vi "config UI.vi"() -> ()   [LabVIEW 2017, in "ScaleAndLimitModule editor node.lvclass"]
doc: "All child modules share this same UI. The UI allows for the configuration of Channels, Parameters, and Error Handling."
uses:
  ScaleAndLimitModule editor node.lvclass
  <vilib>/NI/Configuration Framework/Node/NodeRef.ctl
  <vilib>/NI/Configuration Framework/Node/NISE_CEF_Node.lvclass
  <vilib>/NI/AMC/Message Queue.ctl
  <vilib>/NI/AMC/Message.ctl
  <vilib>/NI/Tools/Keyed Array/KeyedArray.ctl
  <vilib>/NI/Configuration Framework/Node/UserEventRef.ctl
  <vilib>/NI/Configuration Framework/Controls/EventCluster.ctl
  <vilib>/NI/DCAF/Tag Editor Core/control module/configuration/error classification setting.ctl
  <vilib>/NI/Tag Bus Module Framework/runtime/error classification.ctl
  <vilib>/NI/Configuration Framework/Node/RefreshUIEvent.ctl
  <vilib>/NI/Configuration Framework/Node/CacheState.ctl
  <vilib>/NI/Configuration Framework/Node/StopEvent.ctl
  <vilib>/NI/Configuration Framework/Node/NodeChangeEvent.ctl
  <vilib>/NI/DCAF/Tag Editor Core/Table API/Available Tag Menu/channel action event.ctl
  <vilib>/NI/DCAF/Tag Editor Core/Table API/Available Tag Menu/dialog output action.ctl
  <vilib>/NI/Tag Bus Module Framework/channel/TBM channel.lvclass
  <vilib>/NI/Tag Bus/tag/tag descriptor.lvclass
  <vilib>/NI/DCAF/Tag Editor Core/Table API/Table Manager/Call Back Ref Type Def.ctl
  <vilib>/NI/DCAF/Tag Editor Core/Configuration Editor/Classes/Engine Parent/Engine Parent Editor Node.lvclass
  <vilib>/NI/DCAF/Tag Editor Core/Configuration Editor/Classes/Module editor node/module editor node.lvclass
  C:/Program Files (x86)/National Instruments/LabVIEW 2017/vi.lib/NI/Configuration Framework/serializable node/NISE_CEF_serializable node.lvclass
  <vilib>/NI/DCAF/Tag Editor Core/Table API/Table Manager/references.ctl
  <vilib>/NI/DCAF/Tag Editor Core/Table API/Table Manager/Menu Definition.ctl
  <vilib>/NI/DCAF/Tag Editor Core/Table API/Table Manager/Menu Options.ctl
  <vilib>/NI/DCAF/Tag Editor Core/control module/configuration/control module configuration.lvclass
  C:/Program Files (x86)/National Instruments/LabVIEW 2017/vi.lib/NI/Configuration Framework/serializable configuration/NISE_CEF_serializable configuration.lvclass
  <vilib>/NI/DCAF/Tag Editor Core/control module/editor node/control module editor.lvclass
  module/configuration/ScaleAndLimitModule configuration.lvclass
  C:/Program Files (x86)/National Instruments/LabVIEW 2017/vi.lib/NI/DCAF/Tag Editor Core/control module/configuration/control module configuration.lvclass
  C:/Program Files (x86)/National Instruments/LabVIEW 2017/vi.lib/NI/Tag Bus Module Framework/module configuration/TBM module configuration.lvclass
  module/configuration/ScaleAndLimitModule configuration.lvclass/ScaleAndLimitModule configuration.ctl
  <vilib>/NI/DCAF/Tag Editor Core/control module/configuration/control module configuration.lvclass/control module configuration.ctl
  <vilib>/NI/Configuration Framework/serializable configuration/NISE_CEF_serializable configuration.lvclass/NISE_CEF_serializable configuration.ctl
  <vilib>/NI/Tag Bus Module Framework/channel/channel classification.ctl
  module/configuration/Read ScaleAndLimitConfig.vi
  module/configuration/Write ScaleAndLimitConfig.vi
  <vilib>/NI/DCAF/Tag Editor Core/control module/configuration/Write error classifications.vi
  <vilib>/NI/Tag Bus Module Framework/module configuration/TBM module configuration.lvclass
  <vilib>/NI/DCAF/Tag Editor Core/Configuration Editor/Classes/Module editor node/Read Module Configuration.vi
  <vilib>/NI/DCAF/Tag Editor Core/control module/editor node/read fixed channel configuration.vi
  <vilib>/Utility/LVClass/Get LV Class Name.vi
  <vilib>/NI/Configuration Framework/error generator/NISE_error generator.vi
  <vilib>/NI/DCAF/Tag Editor Core/Configuration Editor/Classes/Module editor node/Write Module Configuration.vi
  <vilib>/NI/Configuration Framework/serializable configuration/NISE_CEF_serializable configuration.lvclass
  <vilib>/NI/DCAF/Tag Editor Core/Table API/Listbox/Multi Column Listbox.lvclass
  <vilib>/NI/Configuration Framework/NISE_CEF_TreeControl.lvlib
  <vilib>/NI/DCAF/Tag Editor Core/Table API/Table Manager.lvlib
  <vilib>/NI/DCAF UI Toolkit/Controls/DCAF UI Elements.lvlib
  <vilib>/NI/Tools/Keyed Array/Tools_KeyedArray.lvlib
  <vilib>/NI/AMC/AMC.lvlib
  <vilib>/NI/DCAF/Tag Editor Core/Table API/Table Manager/Table Manager.lvclass
  <vilib>/NI/Tag Bus Module Framework/runtime/TBM module execution interface.lvclass
panel:
  in  "Enum":i32
  in  "user event out":refnum<user-event>
  in  "Top Level Tab Control":T1(tab)
  in  "Values":T2(array[cluster])
  in  "Channels Listbox":i32(listbox)
  in  "mapall":bool
  in  "mapwriters":bool
  in  "Parameters Listbox":i32(listbox)
  in  "error classifications":T3[](array[typedef])
  in  "node change":T5
  in  "stop event":T6
  in  "cache state":T7
  in  "refresh UI":T8
  in  "user event":T9
  in  "main queue":T10
  in  "node ref":T11
  # "Name                                       M                                 B                      High Limit                 Low Limit            Limits Enable"
  # "Y=M*(X-B)"
  # "0"
  # "5"
  # "10"
  # "15"
  # "(Single-Click to Edit)"
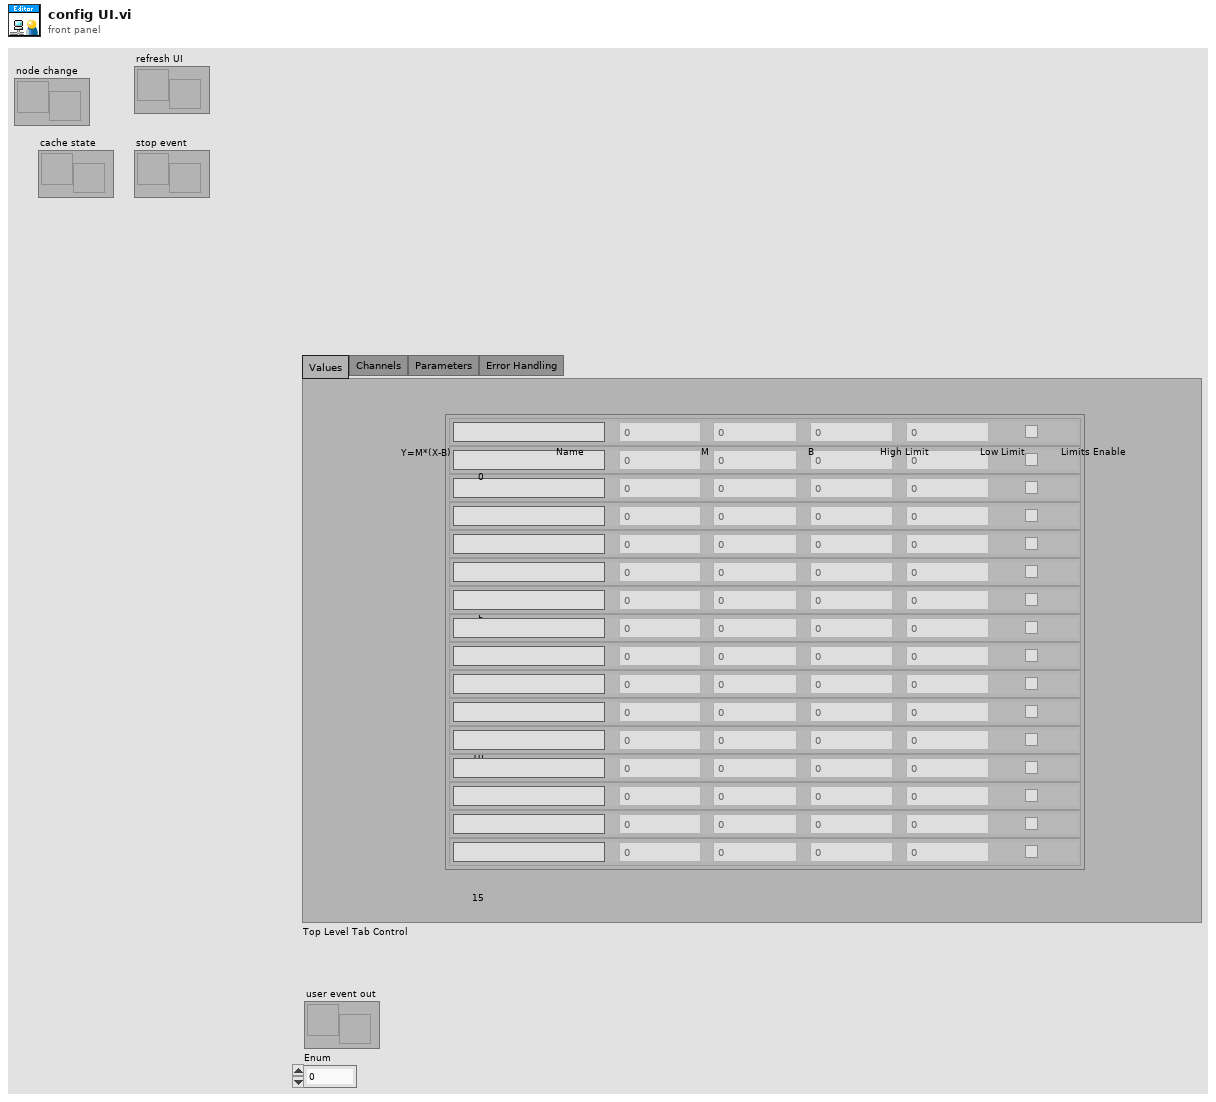
[diagram p1: front panel]
types:
  T1 = enum32{"Values", "Channels", "Parameters", "Error Handling"}
  T2 = cluster{"Name":string, "M":sgl, "B":i16, "HighLimit":sgl, "LowLimit":sgl, "LimitsEnabled":bool}[]
  T3 = typedef "control module configuration.lvclass/error classification setting.ctl" = cluster{"code":i32, "error classification":T4}
  T4 = typedef "TBM module execution interface.lvclass/error classification.ctl" = enum16{"unknown", "none", "trivial", "recoverable", "critical"}
  T5 = typedef "NISE_CEF_Node.lvclass/NodeChangeEvent.ctl" = refnum<user-event>
  T6 = typedef "NISE_CEF_Node.lvclass/StopEvent.ctl" = refnum<user-event>
  T7 = typedef "NISE_CEF_Node.lvclass/CacheState.ctl" = refnum<user-event>
  T8 = typedef "NISE_CEF_Node.lvclass/RefreshUIEvent.ctl" = refnum<user-event>
  T9 = typedef "NISE_CEF_Node.lvclass/UserEventRef.ctl" = refnum<user-event>
  T10 = typedef "AMC.lvlib/Message Queue.ctl" = refnum<queue>
  T11 = typedef "NISE_CEF_Node.lvclass/NodeRef.ctl" = refnum<data-value>
  T12 = typedef "Table Manager.lvlib/Table Manager.lvclass/Menu Definition.ctl" = cluster{"Menu Name":string, "Menu Options":T13}
  T13 = typedef "Table Manager.lvlib/Table Manager.lvclass/Menu Options.ctl" = enum16{"Always Show", "Show When Used", "Show When Empty"}
  T14 = typedef "Table Manager.lvlib/Table Manager.lvclass/references.ctl" = cluster{"stop event":T6, "refresh UI":T8, "cache state":T7, "node change":T5, "user event out":refnum<user-event>, "main queue":T10, "user event":T9}
  T15 = typedef "Table Manager.lvlib/Column.lvclass/Column Descriptor.ctl" = cluster{"name":string, "caption":string, "Column Type":T16, "Params":string, "AutoSizeMode":i32, "FillWeight":sgl, "MinWidth":u32, "tooltip":string, "Enum Reference":refnum<vi>, "Channel suffix":string, "Read Only":bool, "Call Back VI":T17, "DT Dependency":i32, "name dependency":i32, "data type":T18, "Custom Column":refnum<class "Column.lvclass">}
  T16 = typedef "Table Manager.lvlib/Column.lvclass/Column Type.ctl" = enum16{"String", "Mapping", "Enum", "Custom"}
  T17 = typedef "Table Manager.lvlib/Table Manager.lvclass/Call Back Ref Type Def.ctl" = refnum<vi>
  T18 = typedef "tag bus.lvlib/tag descriptor.lvclass/Data Type.ctl" = enum16{"Double", "Single", "I64", "I32", "I16", "I8", "U64", "U32", "U16", "U8", "Boolean", "String", "Array of Double", "Array of Single", "Array of I64", "Array of I32", "Array of I16", "Array of I8", "Array of U64", "Array of U32", "Array of U16", "Array of U8", "Array of Boolean", "Array of String"}
  T19 = typedef "Table Manager.lvlib/Table Manager.lvclass/object ref.ctl" = cluster{"engine":refnum<data-value>, "Node Ref":refnum<data-value>}
  T20 = typedef "Table Manager.lvlib/Table Manager.lvclass/Table Events.ctl" = cluster{"Menu Selection":refnum<user-event>}
  T21 = typedef "NISE_CEF_TreeControl.lvlib/EventCluster.ctl" = cluster{"command":string, "data":string}
  T22 = typedef "ScaleAndLimitInterface.lvlib/Configuration.ctl" = cluster{"Name":string, "M":dbl, "B":i16, "HighLimit":dbl, "LowLimit":dbl, "LimitsEnabled":bool}
  T23 = typedef "TBM channel.lvclass/channel classification.ctl" = enum16{"input data", "output data", "processing parameter", "processing result"}
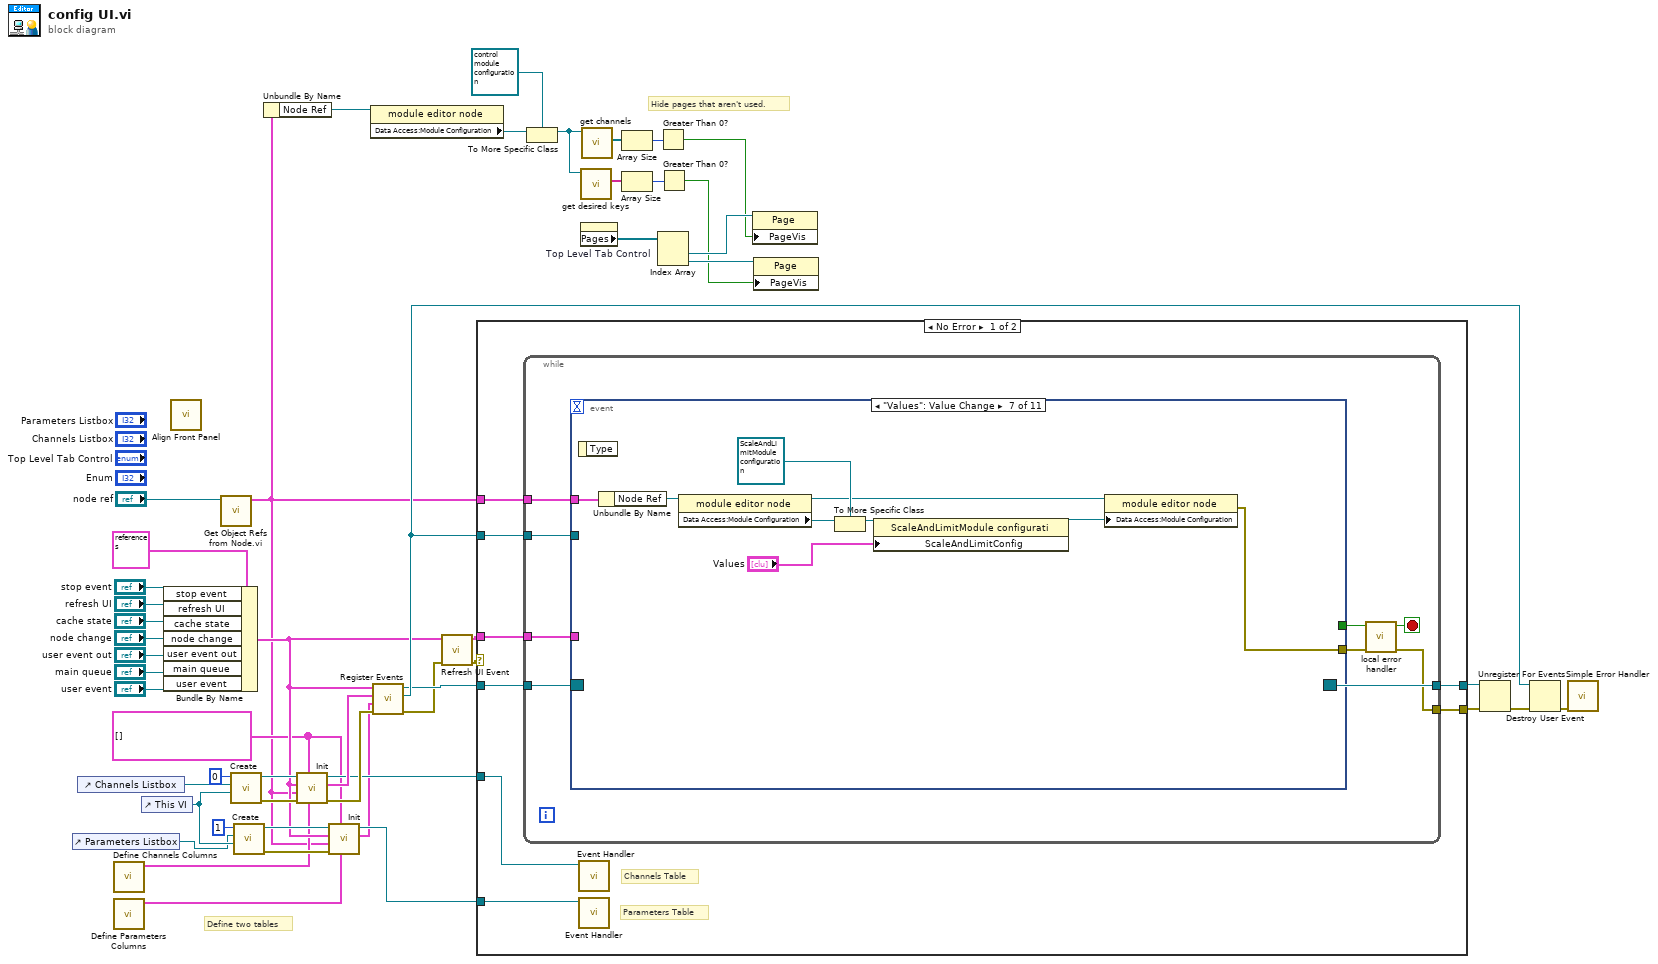
[diagram p0: block diagram]
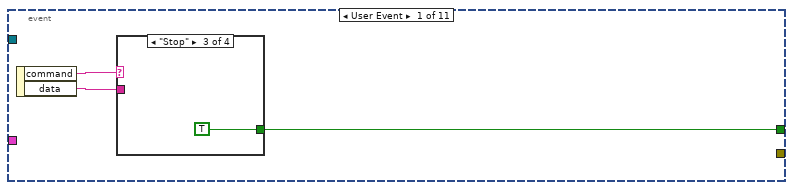
[diagram p2: hidden frame]
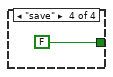
[diagram p5: hidden frame]
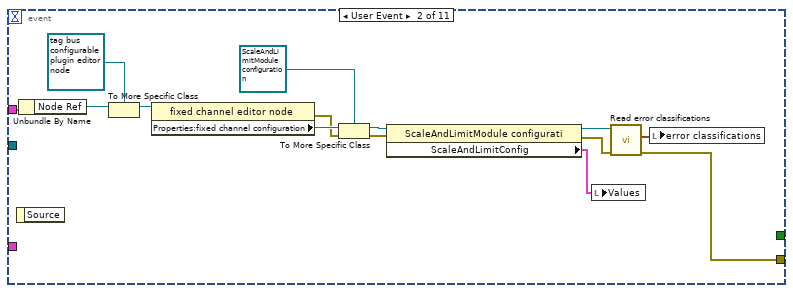
[diagram p6: hidden frame]
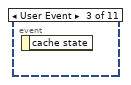
[diagram p7: hidden frame]
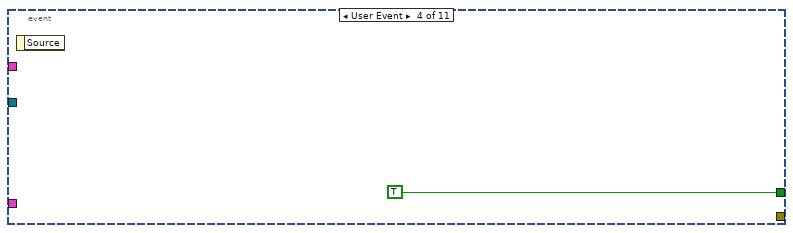
[diagram p8: hidden frame]
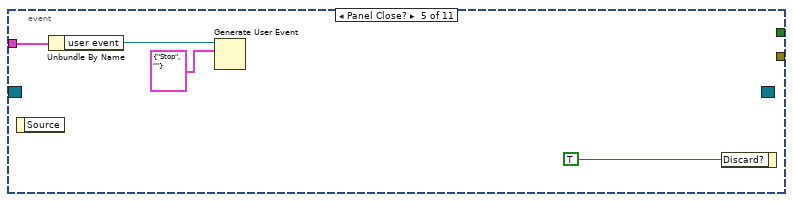
[diagram p9: hidden frame]
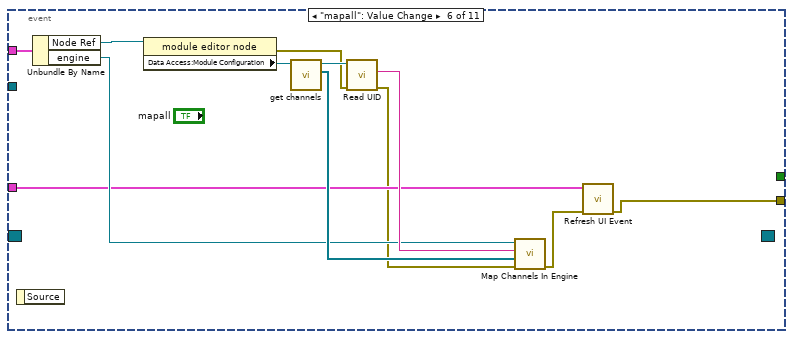
[diagram p10: hidden frame]
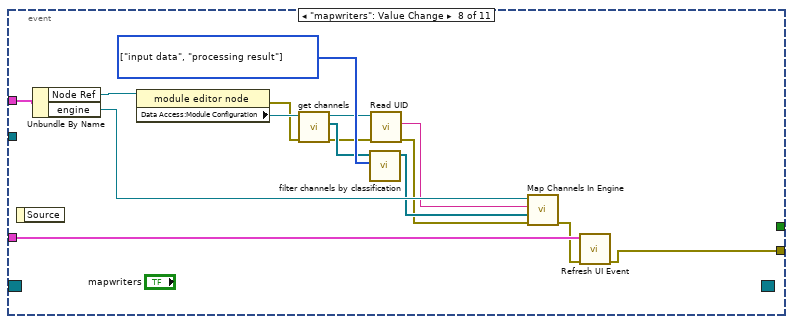
[diagram p11: hidden frame]
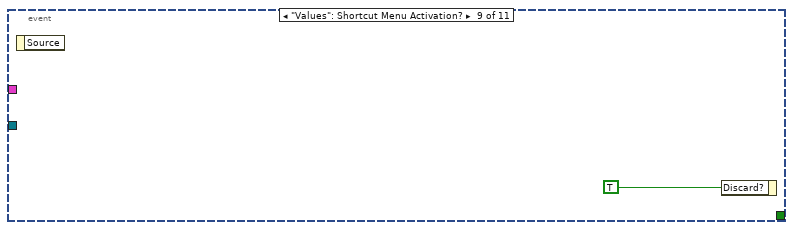
[diagram p12: hidden frame]
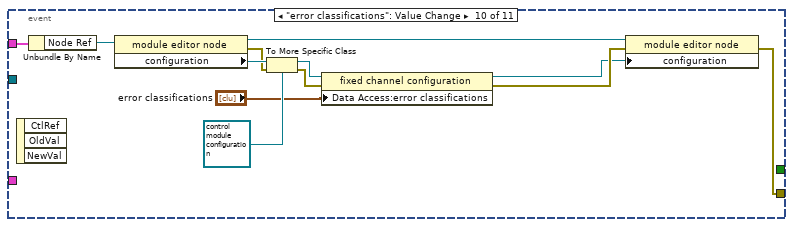
[diagram p13: hidden frame]
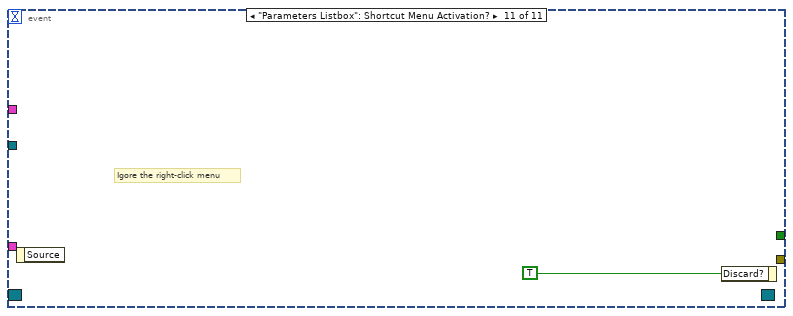
[diagram p14: hidden frame]
diagram:
  w15 = T12[] [] ("Right-Click Menu")
  # "Define two tables"
  # "Hide pages that aren't used."
  n1 = control-ref of="Parameters Listbox"() -> (w18:refnum<vi>)
  n2 = control-ref of="Channels Listbox"() -> (w26:refnum<vi>)
  n3 = call <vilib>:"Define Channels Columns.vi"() -> ("Column Descriptors"=w17:T15[])  [unwired: 11 in]
  n4 = call <vilib>:"Define Parameters Columns.vi"() -> ("Column Descriptors"=w16:T15[])  [unwired: 11 in]
  n5 = control-ref of="This VI"() -> (w22:refnum<vi>)
  n6 = Bundle By Name(cluster=T14 {"stop event"=refnum, "refresh UI"=refnum, "cache state"=refnum, "node change"=refnum, "user event out"=refnum, "main queue"=refnum, "user event"=refnum} ("Event References"), "stop event"="stop event", "refresh UI"="refresh UI", "cache state"="cache state", "node change"="node change", "user event out"="user event out", "main queue"="main queue", "user event"="user event") -> (w19:T14)
  n7 = call <vilib>:"Align Front Panel.vi"() -> ()  [unwired: 10 in, 2 out]
  n8 = call <vilib>:"Get Object Refs from Node.vi.vi"("node ref"="node ref") -> ("Node object refs"=w7:T19)  [unwired: 9 in, 1 out]
  n9 = call <vilib>:"Create.vi"("Top VI"=w22, "Listbox"=w26, "Index"=0) -> ("error out"=w29:errorcluster, "reference out"=w30:refnum<class "Multi Column Listbox.lvclass">)  [unwired: 7 in]
  n10 = call <vilib>:"Create.vi"("Top VI"=w22, "Listbox"=w18, "Index"=1) -> ("error out"=w25:errorcluster, "reference out"=w24:refnum<class "Multi Column Listbox.lvclass">)  [unwired: 7 in]
  n11 = Unbundle By Name(w7) -> ("Node Ref"=w5:refnum<data-value>)
  n12 = call-dynamic "Init.vi"("Column Descriptors"=w17, "Right-Click Menu"=w15, "error in (no error)"=w29, "Node object refs"=w7, "Event References"=w19, "Multi Column Listbox in"=w30) -> ("error out"=w28:errorcluster, "Table Events"=w40:T20, "Multi Column Listbox out"=w27:refnum<class "Multi Column Listbox.lvclass">)  [unwired: 3 in]
  n13 = call-dynamic "Init.vi"("Column Descriptors"=w16, "Right-Click Menu"=w15, "error in (no error)"=w25, "Node object refs"=w7, "Event References"=w19, "Multi Column Listbox in"=w24) -> ("Table Events"=w20:T20, "Multi Column Listbox out"=w21:refnum<class "Multi Column Listbox.lvclass">)  [unwired: 3 in, 1 out]
  n14 = property class="module editor node"(reference=w5) -> ("Data Access:Module Configuration"=w6:refnum<class "TBM module configuration.lvclass">)  [unwired: 1 in, 2 out]
  n15 = call <vilib>:"Register Events.vi"("error in (no error)"=w28, "Parameters Table Events"=w20, "Channels Table Events"=w40, "Event References"=w19) -> ("error out"=w33:errorcluster, "Channel Action"=w39:refnum<user-event>, "Event Registration Refnum"=w38:refnum<event-registration>)  [unwired: 5 in]
  n16 = call <vilib>:"Refresh UI Event.vi"("error in (no error)"=w33, "Event References"=w19) -> ("error out"=w34:errorcluster, "Event References out"=w32:T14)  [unwired: 8 in]
  n17 = case shown="No Error" w34 {
    selector: w34 -> [_ w142]
    tunnel: w38 -> [w58 w141]
    tunnel: [w57 w141] -> w50
    tunnel: [w55 w142] -> w49
    tunnel: w39 -> [w56 _]
    tunnel: w7 -> [w54 _]
    tunnel: w32 -> [w53 _]
    tunnel: w27 -> [w52 _]
    tunnel: w21 -> [w51 _]
    frame No Error {
      # "Parameters Table"
      # "Channels Table"
      n18 = while {
        tunnel: w58 -> [w67]
        tunnel: [w66] -> w57
        tunnel: w56 -> [w65]
        tunnel: [w61] -> w55
        tunnel: w54 -> [w60]
        tunnel: w53 -> [w59]
        stop <- w63 stop-if-true
        n19 = event shown="[6] \"Values\": Value Change" {
          selector: w67 -> [_ _ _ _ _ _ _ _ _ _ _]
          dyn-events: [_ _ _ _ _ _ _ _ _ _ _] -> w66
          timeout: _ -> [_ _ _ _ _ _ _ _ _ _ _]
          tunnel: [w70 _ _ TRUE _ _ _ _ _ _ _] -> w64
          tunnel: [_ w83 _ _ _ w97 w104 w122 _ w139 _] -> w62
          tunnel: w65 -> [_ _ _ _ _ _ _ _ _ _ _]
          tunnel: w60 -> [_ w86 _ _ _ w101 w110 w123 _ w138 _]
          tunnel: w59 -> [_ _ _ _ w89 w96 _ w121 _ _ _]
          event User Event {
            n20 = event-data() -> ("command"=w69:string, "data"=w68:string)  [unwired: 1 in]
            n21 = case shown="\"Stop\"" w69 {
              tunnel: [_ _ TRUE FALSE] -> w70
              tunnel: w68 -> [_ _ _ _]
              frame Default {
              }
              frame "Refresh" {
              }
              frame "Stop" {
              }
              frame "save" {
              }
            }
          }
          event User Event {
            n22 = event-data() -> ()  [unwired: 1 in, 1 out]
            n23 = Unbundle By Name(w86) -> ("Node Ref"=w84:refnum<data-value>)
            n24 = To More Specific Class(target class=refnum<data-value> refnum ("data value reference"), reference=w84) -> (specific class reference=w82:refnum<data-value>)  [unwired: 1 in, 1 out]
            n25 = property class="fixed channel editor node"(reference=w82) -> (error out=w79:errorcluster, "Properties:fixed channel configuration"=w80:refnum<class "control module configuration.lvclass">)  [unwired: 1 in, 1 out]
            n26 = To More Specific Class(target class=refnum<class "ScaleAndLimitModule configuration.lvclass"> refnum ("ScaleAndLimitModule configuration"), reference=w80, error in=w79) -> (specific class reference=w77:refnum<class "ScaleAndLimitModule configuration.lvclass">, error out=w75:errorcluster)
            n27 = property class="ScaleAndLimitModule configurati"(reference=w77, error in=w75) -> (reference out=w76:refnum<class "ScaleAndLimitModule configuration.lvclass">, error out=w74:errorcluster, "ScaleAndLimitConfig"=w73:T22[])
            n28 = local write "Values"(w73) -> ()
            n29 = call <vilib>:"Read error classifications.vi"("error in"=w74, "control module configuration in"=w76) -> ("error out"=w83:errorcluster, "error classifications"=w81:T3[])  [unwired: 7 in, 1 out]
            n30 = local write "error classifications"(w81) -> ()
          }
          event User Event {
            n31 = event-data() -> ()  [unwired: 1 in, 1 out]
          }
          event User Event {
            n32 = event-data() -> ()  [unwired: 1 in, 1 out]
          }
          event Panel Close? {
            n33 = event-data() -> ()  [unwired: 1 in, 1 out]
            n34 = Unbundle By Name(w89) -> ("user event"=w88:T9)
            n35 = Generate User Event(user event=w88, event data cluster=T21 {"command"="Stop", "data"=""} ("event data")) -> ()  [unwired: 2 in, 2 out]
            n36 = event-data("Discard?"=TRUE) -> ()  [unwired: 1 in, 1 out]
          }
          event "mapall": Value Change {
            n37 = event-data() -> ()  [unwired: 1 in, 1 out]
            n38 = Unbundle By Name(w101) -> ("Node Ref"=w100:refnum<data-value>, "engine"=w99:refnum<data-value>)
            n39 = property class="module editor node"(reference=w100) -> (error out=w93:errorcluster, "Data Access:Module Configuration"=w95:refnum<class "TBM module configuration.lvclass">)  [unwired: 1 in, 1 out]
            n40 = call-dynamic "get channels.vi"("module configuration in"=w95) -> ("channels"=w103:refnum<class "TBM channel.lvclass">[], "module configuration out"=w94:refnum<class "TBM module configuration.lvclass">)  [unwired: 9 in]
            n41 = call <vilib>:"Read UID.vi"("error in"=w93, "configuration in"=w94) -> ("error out"=w92:errorcluster, "instance id"=w102:string)  [unwired: 7 in, 1 out]
            n42 = call <vilib>:"Map Channels In Engine.vi"("error in (no error)"=w92, "channels"=w103, "instance id"=w102, "Engine DVR"=w99) -> ("error out"=w98:errorcluster)  [unwired: 7 in]
            n43 = call <vilib>:"Refresh UI Event.vi"("error in (no error)"=w98, "Event References"=w96) -> ("error out"=w97:errorcluster)  [unwired: 8 in, 1 out]
          }
          event "Values": Value Change {
            n44 = event-data() -> ()  [unwired: 1 in, 1 out]
            n45 = Unbundle By Name(w110) -> ("Node Ref"=w111:refnum<data-value>)
            n46 = property class="module editor node"(reference=w111) -> (reference out=w106:refnum<data-value>, "Data Access:Module Configuration"=w112:refnum<class "TBM module configuration.lvclass">)  [unwired: 1 in, 1 out]
            n47 = To More Specific Class(target class=refnum<class "ScaleAndLimitModule configuration.lvclass"> refnum ("ScaleAndLimitModule configuration"), reference=w112) -> (specific class reference=w108:refnum<class "ScaleAndLimitModule configuration.lvclass">)  [unwired: 1 in, 1 out]
            n48 = property class="ScaleAndLimitModule configurati"(reference=w108, "ScaleAndLimitConfig"="Values") -> (reference out=w105:refnum<class "ScaleAndLimitModule configuration.lvclass">)  [unwired: 1 in, 1 out]
            n49 = property class="module editor node"(reference=w106, "Data Access:Module Configuration"=w105) -> (error out=w104:errorcluster)  [unwired: 1 in, 1 out]
          }
          event "mapwriters": Value Change {
            w126 = T23[] [enum."input data", enum."processing result"] items=["input data", "output data", "processing parameter", "processing result"] ("allowed classifications")
            n50 = event-data() -> ()  [unwired: 1 in, 1 out]
            n51 = Unbundle By Name(w123) -> ("Node Ref"=w124:refnum<data-value>, "engine"=w120:refnum<data-value>)
            n52 = property class="module editor node"(reference=w124) -> (error out=w113:errorcluster, "Data Access:Module Configuration"=w115:refnum<class "TBM module configuration.lvclass">)  [unwired: 1 in, 1 out]
            n53 = call-dynamic "get channels.vi"("module configuration in"=w115) -> ("channels"=w125:refnum<class "TBM channel.lvclass">[], "module configuration out"=w114:refnum<class "TBM module configuration.lvclass">)  [unwired: 9 in]
            n54 = call <vilib>:"filter channels by classification.vi"("allowed classifications"=w126, "channels in"=w125) -> ("channels out"=w118:refnum<class "TBM channel.lvclass">[])  [unwired: 9 in]
            n55 = call <vilib>:"Read UID.vi"("error in"=w113, "configuration in"=w114) -> ("error out"=w117:errorcluster, "instance id"=w119:string)  [unwired: 7 in, 1 out]
            n56 = call <vilib>:"Map Channels In Engine.vi"("error in (no error)"=w117, "channels"=w118, "instance id"=w119, "Engine DVR"=w120) -> ("error out"=w116:errorcluster)  [unwired: 7 in]
            n57 = call <vilib>:"Refresh UI Event.vi"("error in (no error)"=w116, "Event References"=w121) -> ("error out"=w122:errorcluster)  [unwired: 8 in, 1 out]
          }
          event "Values": Shortcut Menu Activation? {
            n58 = event-data() -> ()  [unwired: 1 in, 1 out]
            n59 = event-data("Discard?"=TRUE) -> ()  [unwired: 1 in, 1 out]
          }
          event "error classifications": Value Change {
            n60 = event-data() -> ()  [unwired: 1 in, 3 out]
            n61 = Unbundle By Name(w138) -> ("Node Ref"=w133:refnum<data-value>)
            n62 = property class="module editor node"(reference=w133) -> (reference out=w137:refnum<data-value>, error out=w129:errorcluster, "configuration"=w132:refnum<class "NISE_CEF_serializable configuration.lvclass">)  [unwired: 1 in]
            n63 = To More Specific Class(target class=refnum<class "control module configuration.lvclass"> refnum ("fixed channel configuration"), reference=w132, error in=w129) -> (specific class reference=w134:refnum<class "control module configuration.lvclass">, error out=w128:errorcluster)
            n64 = property class="fixed channel configuration"(reference=w134, error in=w128, "Data Access:error classifications"="error classifications") -> (reference out=w135:refnum<class "control module configuration.lvclass">, error out=w136:errorcluster)
            n65 = property class="module editor node"(reference=w137, error in=w136, "configuration"=w135) -> (error out=w139:errorcluster)  [unwired: 1 out]
          }
          event "Parameters Listbox": Shortcut Menu Activation? {
            # "Igore the right-click menu"
            n66 = event-data() -> ()  [unwired: 1 in, 1 out]
            n67 = event-data("Discard?"=TRUE) -> ()  [unwired: 1 in, 1 out]
          }
        }
        n68 = call <vilib>:"local error handler.vi"("error in (no error)"=w62, "Stop in"=w64) -> ("error out"=w61:errorcluster, "Stop out"=w63:bool)  [unwired: 8 in]
      }
      n69 = call-dynamic "Event Handler.vi"("Listbox in"=w52) -> ()  [unwired: 9 in, 2 out]
      n70 = call-dynamic "Event Handler.vi"("Listbox in"=w51) -> ()  [unwired: 9 in, 2 out]
    }
    frame Error {
    }
  }
  n71 = To More Specific Class(target class=refnum<class "control module configuration.lvclass"> refnum ("fixed channel configuration"), reference=w6) -> (specific class reference=w3:refnum<class "control module configuration.lvclass">)  [unwired: 1 in, 1 out]
  n72 = call-dynamic "get desired keys.vi"("fixed channel configuration in"=w3) -> ("desired keys"=w11:string[])  [unwired: 8 in, 2 out]
  n73 = property on="Top Level Tab Control" class="TabCtl (strict)"() -> ("Pages"=w8:refnum<vi>[])  [unwired: 2 in, 2 out]
  n74 = call-dynamic "get channels.vi"("fixed channel configuration in"=w3) -> ("channels"=w14:refnum<class "TBM channel.lvclass">[])  [unwired: 9 in, 1 out]
  n75 = Array Size(array=w14) -> (size(s)=w13:i32)
  n76 = Array Size(array=w11) -> (size(s)=w12:i32)
  n77 = Greater Than 0?(x=w13) -> (x > 0?=w2:bool)
  n78 = Index Array(array=w8) -> (element #1=w9:refnum<vi>, element #2=w10:refnum<vi>)  [unwired: 2 in]
  n79 = Greater Than 0?(x=w12) -> (x > 0?=w1:bool)
  n80 = property class="Page"(reference=w9, "PageVis"=w2) -> ()  [unwired: 1 in, 2 out]
  n81 = property class="Page"(reference=w10, "PageVis"=w1) -> ()  [unwired: 1 in, 2 out]
  n82 = Unregister For Events(event registration refnum=w50, error in=w49) -> (error out=w48:errorcluster)
  n83 = Destroy User Event(user event=w39, error in=w48) -> (error out=w47:errorcluster)
  n84 = call <vilib>:"Simple Error Handler.vi"("error in (no error)"=w47) -> ()  [unwired: 4 in, 5 out]
